vi "getpointagebyuserid.vi"(1 "id":dbl, 2 "Fichier DB":string) -> (0 "Données pointage":string[][](table))   [LabVIEW 2024]
uses:
  <vilib>/drjdpowell/SQLite Library/SQL Connection/Open (string).vi
  <vilib>/drjdpowell/SQLite Library/SQL Connection/Execute SQL.vi
  <vilib>/drjdpowell/SQLite Library/SQL Connection/Connection.lvclass
  <vilib>/drjdpowell/SQLite Library/SQLite.lvlib
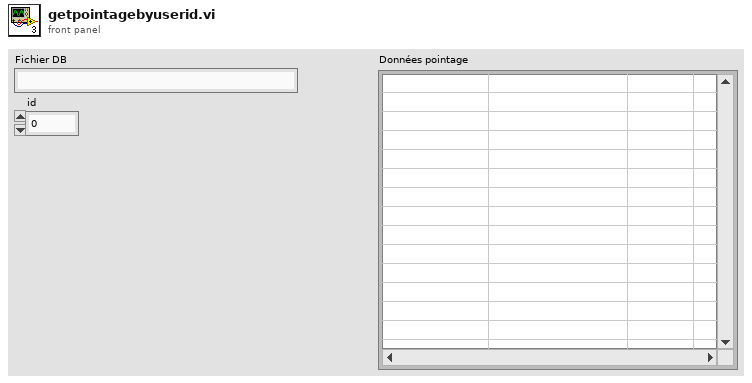
[diagram p1: front panel]
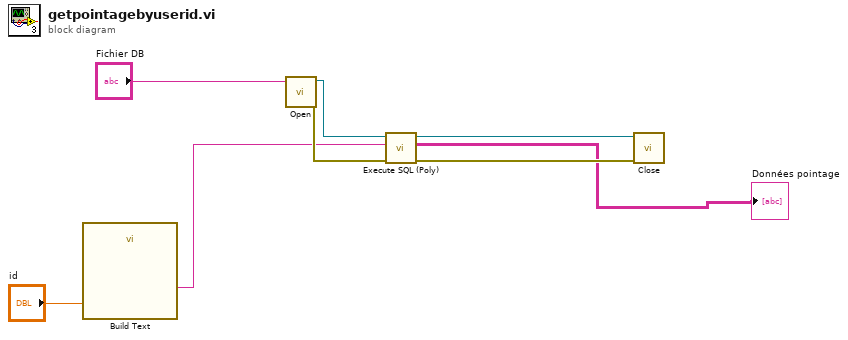
[diagram p0: block diagram]
diagram:
  n1 = call "Build Text"("id"="id") -> ("Result"=w3:string)  [unwired: 13 in, 1 out]
  n2 = call-poly <vilib>:"Open.vi"("db file"="Fichier DB") -> ("error out"=w5:errorcluster, "SQLite Connection"=w6:refnum<class "Connection.lvclass">)  [unwired: 9 in]
  n3 = call-poly <vilib>:"Execute SQL (Poly).vi"("error in (no error)"=w5, "SQL"=w3, "SQLite Connection in"=w6) -> ("error out"=w7:errorcluster, "Result Set"=→"Données pointage":string[][], "SQLite Connection"=w8:refnum<class "Connection.lvclass">)  [unwired: 5 in, 1 out]
  n4 = call-dynamic "Close.vi"("error in (no error)"=w7, "SQLite Connection in"=w8) -> ()  [unwired: 9 in, 1 out]
